vi "PathPlanner_Util_TrajStatesToPathPlannerStates.vi"(11 "TrajStates":T1[](array[typedef]) {"POSE"."ROTATION"."SIN" format="%13.4f"; "POSE"."ROTATION"."COS" format="%13.4f"; "POSE"."ROTATION"."VALUE" format="%13.4f"; "POSE"."TRANSLATION"."Y" format="%14.3f"; "POSE"."TRANSLATION"."X" format="%14.3f"}) -> (3 "PathPlannerStates":T5[](array[typedef]) {"TargetHolonomicRotation"."SIN" format="%13.4f"; "TargetHolonomicRotation"."COS" format="%13.4f"; "TargetHolonomicRotation"."VALUE" format="%13.4f"; "Heading"."SIN" format="%13.4f"; "Heading"."COS" format="%13.4f"; "Heading"."VALUE" format="%13.4f"; "PositionMeters"."Y" format="%14.3f"; "PositionMeters"."X" format="%14.3f"})   [LabVIEW 2019]
uses:
  <vilib>/Rock Robotics/WPI/ThirdParty/JAS_Junk/TrajLib/TypeDef/ROTATION2D.ctl
  <vilib>/Rock Robotics/WPI/ThirdParty/JAS_Junk/TrajLib/Trajectory_Library.lvlib
  <vilib>/Rock Robotics/WPI/ThirdParty/JAS_Junk/TrajLib/TypeDef/TRANSLATION2D.ctl
  <vilib>/Rock Robotics/WPI/ThirdParty/MJansen/PathPlanner/TypeDef/PathPlannerTrajectoryState.ctl
  <vilib>/Rock Robotics/WPI/ThirdParty/MJansen/PathPlanner/PathPlanner24.lvlib
  <vilib>/Rock Robotics/WPI/ThirdParty/MJansen/PathPlanner/TypeDef/PathPlannerPathConstraints.ctl
  <vilib>/Rock Robotics/WPI/ThirdParty/JAS_Junk/TrajLib/TypeDef/POSE2D.ctl
  <vilib>/Rock Robotics/WPI/ThirdParty/JAS_Junk/TrajLib/TypeDef/TRAJ_STATE.ctl
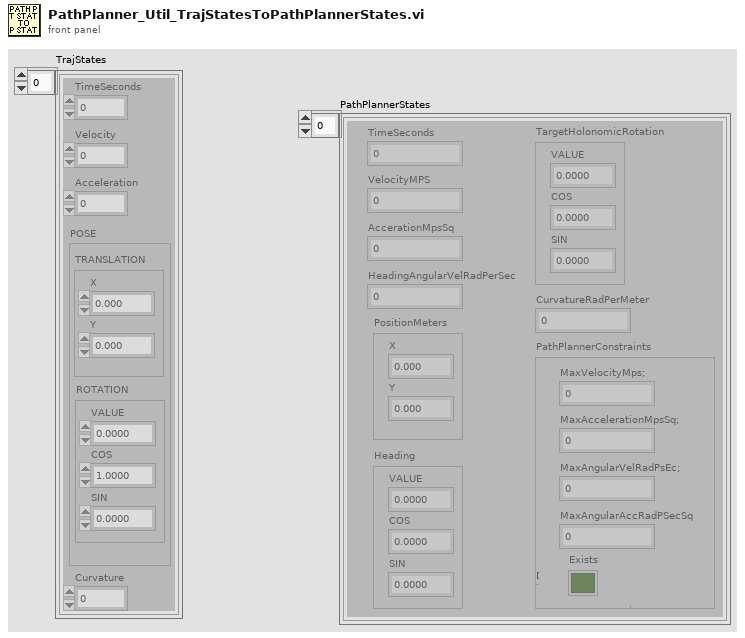
[diagram p1: front panel]
types:
  T1 = typedef "Trajectory_Library.lvlib/TRAJ_STATE.ctl" = cluster{"TimeSeconds":dbl, "Velocity":dbl, "Acceleration":dbl, "POSE":T2, "Curvature":dbl}
  T2 = typedef "Trajectory_Library.lvlib/POSE2D.ctl" = cluster{"TRANSLATION":T3, "ROTATION":T4}
  T3 = typedef "Trajectory_Library.lvlib/TRANSLATION2D.ctl" = cluster{"X":dbl, "Y":dbl}
  T4 = typedef "Trajectory_Library.lvlib/ROTATION2D.ctl" = cluster{"VALUE":dbl, "COS":dbl, "SIN":dbl}
  T5 = typedef "PathPlanner24.lvlib/PathPlannerTrajectoryState.ctl" = cluster{"TimeSeconds":dbl, "VelocityMPS":dbl, "AccerationMpsSq":dbl, "HeadingAngularVelRadPerSec":dbl, "PositionMeters":T3, "Heading":T4, "TargetHolonomicRotation":T4, "CurvatureRadPerMeter":dbl, "DeltaPos":dbl, "PathPlannerConstraints":T6}
  T6 = typedef "PathPlanner24.lvlib/PathPlannerPathConstraints.ctl" = cluster{"MaxVelocityMps;":dbl, "MaxAccelerationMpsSq;":dbl, "MaxAngularVelRadPsEc;":dbl, "MaxAngularAccRadPSecSq":dbl, "Exists":bool}
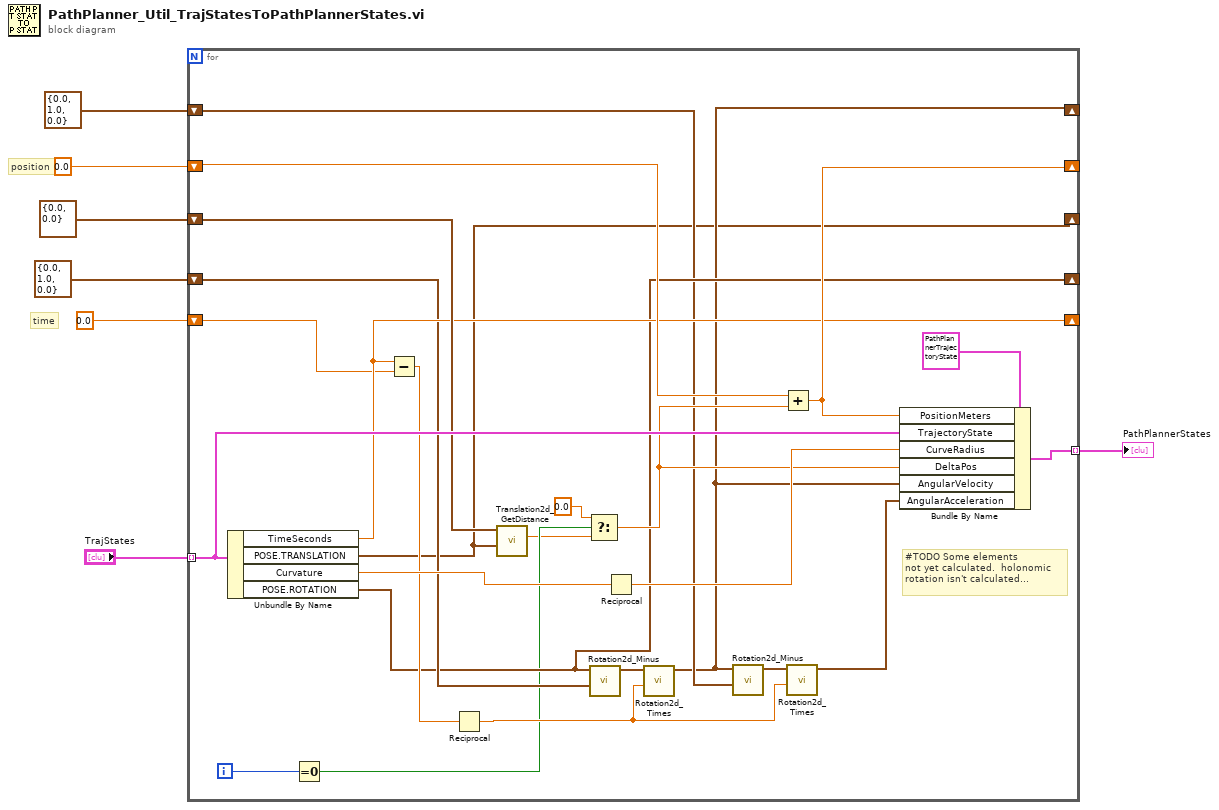
[diagram p0: block diagram]
diagram:
  # "time"
  # "position"
  n1 = for {
    tunnel: "TrajStates" -> [w30] mode=indexing
    tunnel: [w31] -> w7 mode=indexing
    shift-right: [w10] -> _
    shift-left: T3 {"X"=0.0, "Y"=0.0} ("TRANSLATION") -> [w27]
    shift-right: [w23] -> _
    shift-left: 0.0 -> [w24]
    shift-right: [w15] -> _
    shift-left: T4 {"VALUE"=0.0, "COS"=1.0, "SIN"=0.0} ("ROTATION") -> [w16]
    shift-right: [w22] -> _
    shift-left: 0.0 -> [w21]
    shift-right: [w13] -> _
    shift-left: T4 {"VALUE"=0.0, "COS"=1.0, "SIN"=0.0} ("ROTATION") -> [w14]
    i -> [w26]
    # "#TODO Some elements\nnot yet calculated.  holonomic\nrotation isn't calculated..."
    n2 = Unbundle By Name(w30) -> ("TimeSeconds"=w22:dbl, "POSE.TRANSLATION"=w10:T3, "Curvature"=w29:dbl, "POSE.ROTATION"=w15:T4)
    n3 = Equal To 0?(x=w26) -> (x = 0?=w11:bool)
    n4 = Subtract(x=w22, y=w21) -> (x-y=w18:dbl)
    n5 = Reciprocal(x=w18) -> (1/x=w17:dbl)
    n6 = call <vilib>:"Translation2d_GetDistance.vi"("other Translation"=w10, "In Translation"=w27) -> ("Distance"=w9:dbl)  [unwired: 9 in]
    n7 = Select(t=0.0, s=w11, f=w9) -> (s? t:f=w25:dbl)
    n8 = call <vilib>:"Rotation2d_Minus.vi"("other ROTATION"=w16, "in ROTATION"=w15) -> ("out ROTATION"=w20:T4)  [unwired: 9 in]
    n9 = Reciprocal(x=w29) -> (1/x=w28:dbl)
    n10 = call <vilib>:"Rotation2d_Times.vi"("Scalar"=w17, "in ROTATION"=w20) -> ("out ROTATION"=w13:T4)  [unwired: 9 in]
    n11 = call <vilib>:"Rotation2d_Minus.vi"("other ROTATION"=w14, "in ROTATION"=w13) -> ("out ROTATION"=w19:T4)  [unwired: 9 in]
    n12 = Add(x=w24, y=w25) -> (x+y=w23:dbl)
    n13 = call <vilib>:"Rotation2d_Times.vi"("Scalar"=w17, "in ROTATION"=w19) -> ("out ROTATION"=w12:T4)  [unwired: 9 in]
    n14 = Bundle By Name(cluster=T5 {"TimeSeconds"=0.0, "VelocityMPS"=0.0, "AccerationMpsSq"=0.0, "HeadingAngularVelRadPerSec"=0.0, "PositionMeters"={"X"=0.0, "Y"=1.0}, "Heading"={"VALUE"=0.0, "COS"=1.0, "SIN"=0.0}, "TargetHolonomicRotation"={"VALUE"=0.0, "COS"=0.0, "SIN"=0.0}, "CurvatureRadPerMeter"=0.0, "DeltaPos"=0.0, "PathPlannerConstraints"={"MaxVelocityMps;"=0.0, "MaxAccelerationMpsSq;"=1.0, "MaxAngularVelRadPsEc;"=0.0, "MaxAngularAccRadPSecSq"=0.0, "Exists"=FALSE}} ("PathPlannerState"), "PositionMeters"=w23, "TrajectoryState"=w30, "CurveRadius"=w28, "DeltaPos"=w25, "AngularVelocity"=w13, "AngularAcceleration"=w12) -> (w31:T5)
  }
  "PathPlannerStates" <- w7
